vi "IHM_GetNumericValue.vi"(4 "error in (no error)":errorcluster caption="entrée d'erreur (pas d'erreur)", 7 "Ref_IN":T1) -> (0 "Error out":errorcluster, 2 "NumericValue":i32, 3 "Ref_OUT":T1)   [LabVIEW 2013]
panel:
  out "ClassName":string
  out "Name":string
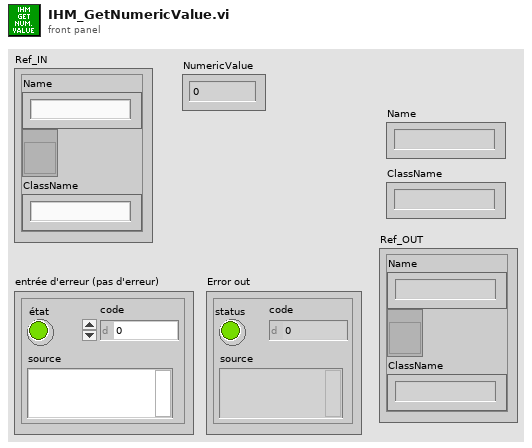
[diagram p1: front panel]
types:
  T1 = cluster{"Name":string, refnum<vi>, "ClassName":string}
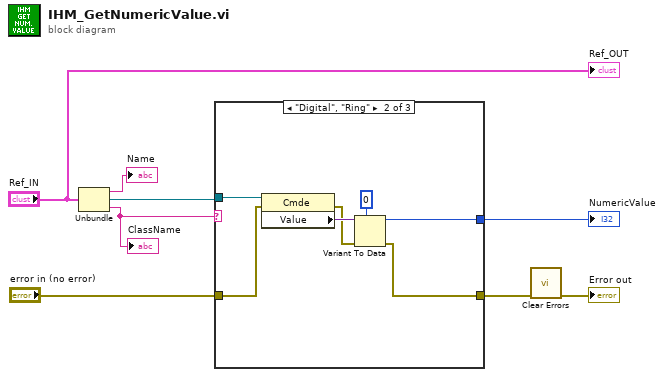
[diagram p0: block diagram]
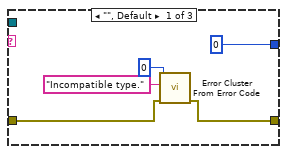
[diagram p2: hidden frame]
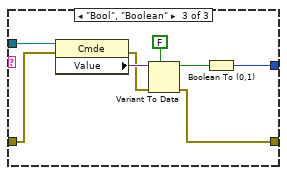
[diagram p3: hidden frame]
diagram:
  n1 = Unbundle("Ref_IN") -> ("Name"=→"Name":string, w7:refnum<vi>, "ClassName"=w8:string)
  "ClassName" <- w8
  n2 = case shown="\"Digital\", \"Ring\"" w8 {
    tunnel: w7 -> [_ w18 w27]
    tunnel: [0 w17 w21] -> w4
    tunnel: "error in (no error)" -> [w12 w16 w26]
    tunnel: [w11 w14 w24] -> w2
    frame "", Default {
      n3 = call <vilib>:"Error Cluster From Error Code.vi"("error in (no error)"=w12, "error message (\"\")"="Incompatible type." ("error message (\"\")"), "error code (0)"=0) -> ("error out"=w11:errorcluster)  [unwired: 6 in]
    }
    frame "Digital", "Ring" {
      n4 = property class="Cmde"(reference=w18, error in=w16) -> (error out=w15:errorcluster, "Value"=w19:variant)  [unwired: 1 out]
      n5 = Variant To Data(error in=w15, type=0, Variant=w19) -> (data=w17:i32, error out=w14:errorcluster)
    }
    frame "Bool", "Boolean" {
      n6 = property class="Cmde"(reference=w27, error in=w26) -> (error out=w25:errorcluster, "Value"=w28:variant)  [unwired: 1 out]
      n7 = Variant To Data(error in=w25, type=FALSE, Variant=w28) -> (data=w22:bool, error out=w24:errorcluster)
      n8 = Boolean To (0,1)(Boolean=w22) -> (0, 1=w21:i16)
    }
  }
  "NumericValue" <- w4
  n9 = call <vilib>:"Clear Errors.vi"("error in (no error)"=w2) -> ("error out"=→"Error out":errorcluster)  [unwired: 6 in]
  "Ref_OUT" <- "Ref_IN"
